vi "Listen for Results.vi"(8 "error in (no error)":errorcluster, 9 "Timeout [ms]":i32=-1, 11 "Icon Decorator In":refnum<class "Icon Decorator.lvclass">) -> (0 "error out":errorcluster, 3 "Icon Decorator Out":refnum<class "Icon Decorator.lvclass">)   [LabVIEW 2020, in "Icon Decorator.lvclass"]
uses:
  Icon Decorator.lvclass
  Icon Decorator.lvclass/Icon Decorator.ctl
  Result Types/Case Result/Private/Merge Status.vi
  Result Types/Case Result/Test Case Result.lvlib
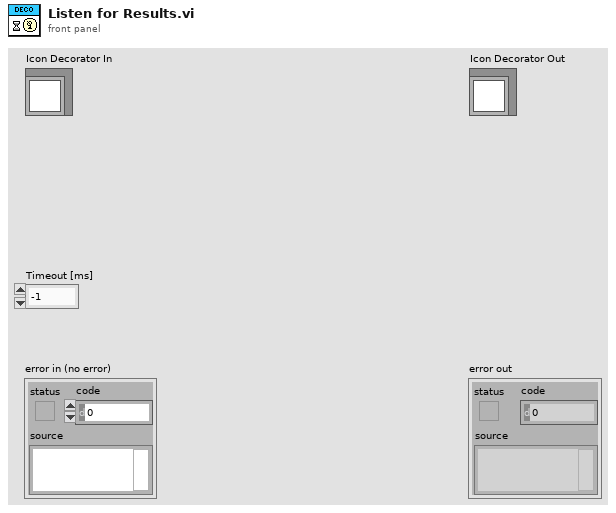
[diagram p1: front panel]
types:
  T1 = cluster{"Test Cases Found Registration":refnum<event-registration>, "Result Events":refnum<event-registration>}
  T2 = typedef "Test Case Result.lvlib/Test Case Result type.ctl" = map{string, T3}
  T3 = typedef "Method Result.lvlib/Method Result type.ctl" = cluster{"Test Case":string, "Test Method Name":string, "Status":T4, "Assertion Results":T5[], "Execution time":dbl, "Result String":string}
  T4 = typedef "Assertion Result.lvlib/Status.ctl" = enum16{"Pass", "Fail", "Error", "Skipped", "Setup Error", "Broken", "Teardown Error"}
  T5 = typedef "Assertion Result.lvlib/Assertion Result type.ctl" = cluster{"Status":T4, "Message":string, "Description":string, "Assertion Type":T6}
  T6 = typedef "Assertion Result.lvlib/Assertion Type.ctl" = enum16{"None", "Pass", "Fail", "Skip", "Pass if Equal", "Fail if Equal", "Pass if Error", "Fail if Error", "Pass if", "Fail if"}
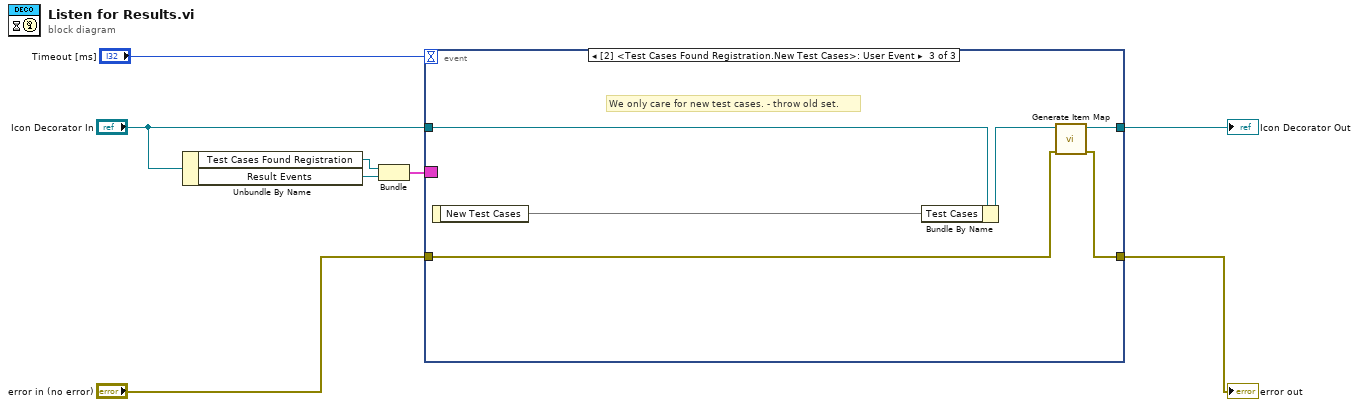
[diagram p0: block diagram]
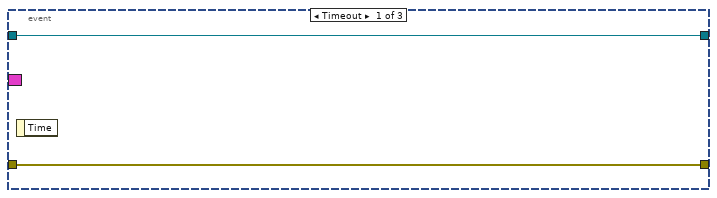
[diagram p2: hidden frame]
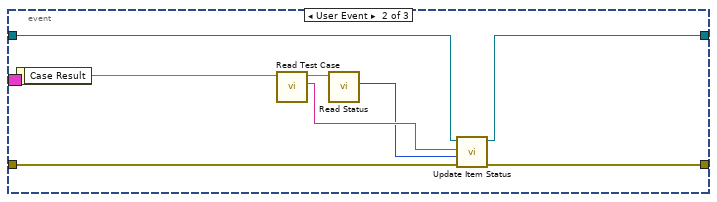
[diagram p3: hidden frame]
diagram:
  n1 = Unbundle By Name("Icon Decorator In") -> ("Test Cases Found Registration"=w2:refnum<event-registration>, "Result Events"=w3:refnum<event-registration>)
  n2 = Bundle("Test Cases Found Registration"=w2, "Result Events"=w3) -> (w4:T1)  [unwired: 1 in]
  n3 = event shown="[2] <Test Cases Found Registration.New Test Cases>: User Event" {
    selector: w4 -> [_ _ _]
    dyn-events: _ -> [_ _ _]
    timeout: "Timeout [ms]" -> [_ _ _]
    tunnel: "error in (no error)" -> [w9 w12 w20]
    tunnel: "Icon Decorator In" -> [w10 w16 w23]
    tunnel: [w10 w13 w24] -> w6
    tunnel: [w9 w17 w21] -> w5
    event Timeout {
      n4 = event-data() -> ()  [unwired: 1 in, 1 out]
    }
    event User Event {
      n5 = event-data() -> ("Case Result"=w11:T2)  [unwired: 1 in]
      n6 = call "Read Test Case.vi"("Test Case Result In"=w11) -> ("Test Case"=w15:string, "Test Case Result Out"=w18:T2)  [unwired: 9 in]
      n7 = call "Read Status.vi"("Test Case Result In"=w18) -> ("Status"=w14:T4)  [unwired: 8 in, 2 out]
      n8 = call "Update Item Status.vi"("error in (no error)"=w12, "Status"=w14, "Test Case"=w15, "Icon Decorator In"=w16) -> ("error out"=w17:errorcluster, "Icon Decorator Out"=w13:refnum<class "Icon Decorator.lvclass">)  [unwired: 6 in]
    }
    event User Event {
      # "We only care for new test cases. - throw old set."
      n9 = event-data() -> ("New Test Cases"=w19:set{path})  [unwired: 1 in]
      n10 = Bundle By Name(cluster=w23, "Test Cases"=w19) -> (w22:refnum<class "Icon Decorator.lvclass">)
      n11 = call "Generate Item Map.vi"("error in (no error)"=w20, "Icon Decorator In"=w22) -> ("error out"=w21:errorcluster, "Icon Decorator Out"=w24:refnum<class "Icon Decorator.lvclass">)  [unwired: 8 in]
    }
  }
  "error out" <- w5
  "Icon Decorator Out" <- w6
